vi "ErrorHandler.vi"(3 "error in":errorcluster) -> (8 "error?":bool, 11 "error out":errorcluster)   [LabVIEW 2020, in "Phidget Common.lvlib"]
doc: "Translates the user-error event codes returned by Phidget VIs into the Phidget error code, and provides a description."
uses:
  <instrlib>/Phidgets/Phidget Common/Phidget Common.lvlib
  <vilib>/Utility/importsl/GetValueByPointer/datatype.ctl
  <vilib>/Utility/importsl/GetValueByPointer/GetValueByPointer.xnode
  phidget22.dll
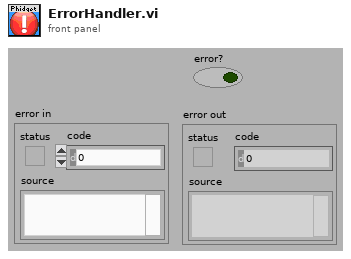
[diagram p1: front panel]
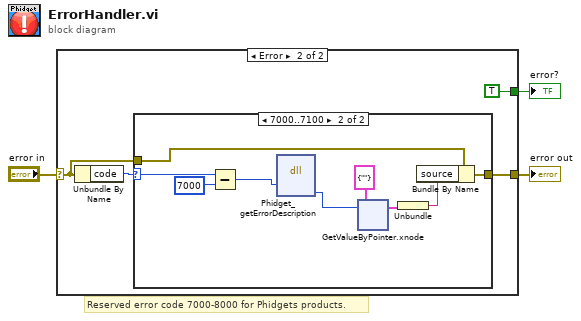
[diagram p0: block diagram]
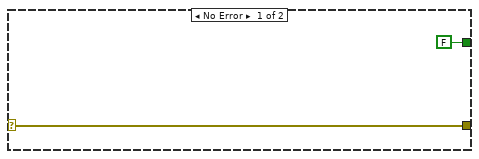
[diagram p2: hidden frame]
diagram:
  # "Reserved error code 7000-8000 for Phidgets products."
  n1 = case shown="Error" "error in" {
    selector: "error in" -> [w5 w9]
    tunnel: [w5 w8] -> w2
    tunnel: [FALSE ("error?") TRUE ("error?")] -> w1
    frame No Error {
    }
    frame Error {
      n2 = Unbundle By Name(w9) -> ("code"=w6:i32)
      n3 = case shown="7000..7100" w6 {
        selector: w6 -> [_ w16]
        tunnel: w9 -> [w10 w19]
        tunnel: [w10 w18] -> w8
        frame 0, Default {
        }
        frame 7000..7100 {
          n4 = Subtract(x=w16, y=7000) -> (x-y=w15:i32)
          n5 = dll-call lib="phidget22.*" fn="Phidget_getErrorDescription"("ErrorCode"=w15) -> ("ErrorMsg"=w14:u64)  [unwired: 6 in, 2 out]
          n6 = xnode "GetValueByPointer.xnode"("Pointer"=w14, "InputType"=cluster{string} {""}) -> ("Output"=w12:cluster{string})  [unwired: 2 in, 1 out]
          n7 = Unbundle(w12) -> (w11:string)
          n8 = Bundle By Name(cluster=w19, "source"=w11) -> (w18:errorcluster)
        }
      }
    }
  }
  "error?" <- w1
  "error out" <- w2
